vi "new destination folder for pictures.vi"(7 "scanners[]":string[](array[string]), 8 "error in":errorcluster, 10 "Info":T1={"Make"="", "Model"="", "Orientation"=0, "Date"=timestamp(0 s since 1904-01-01), "Width"=0, "Height"=0, "Square?"=FALSE, "File Name"="", "Extension"="", "Valid?"=FALSE, "Path"=path "", "size"=0, "No Ext?"=FALSE, "prefix?"=FALSE, "String"="", "Name Type"=enum."Event Sufix"}, 11 "dest path":path) -> (0 "error out":errorcluster, 3 "new dest filder path":path)   [LabVIEW 2023, in "File Classes.lvlib" / "Picture File.lvclass"]
uses:
  Picture File.lvclass
  Controls/exif data cluster.ctl
  Controls/rename type enum.ctl
  File Classes.lvlib
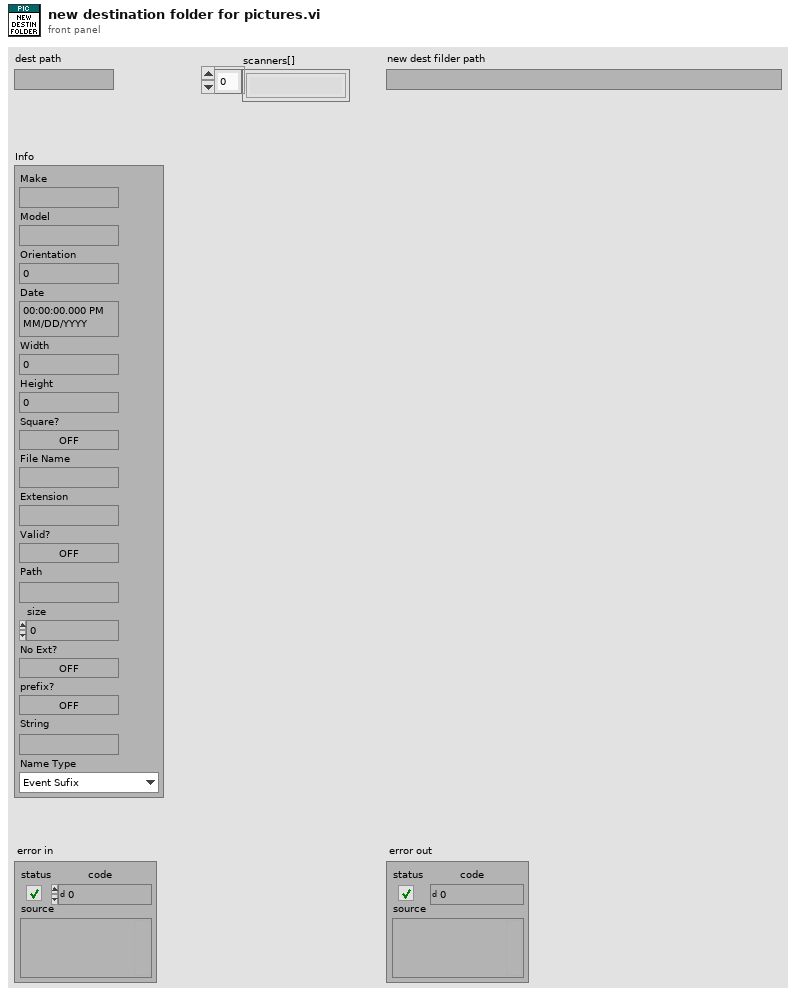
[diagram p1: front panel]
types:
  T1 = typedef "File Classes.lvlib/exif data cluster.ctl" = cluster{"Make":string, "Model":string, "Orientation":u16, "Date":timestamp, "Width":u16, "Height":u16, "Square?":bool, "File Name":string, "Extension":string, "Valid?":bool, "Path":path, "size":i64, "No Ext?":bool, "prefix?":bool, "String":string, "Name Type":T2}
  T2 = typedef "File Classes.lvlib/rename type enum.ctl" = enum16{"Date & Time (Default)", "Model Sufix", "Event Sufix", "Model & Event Sufix"}
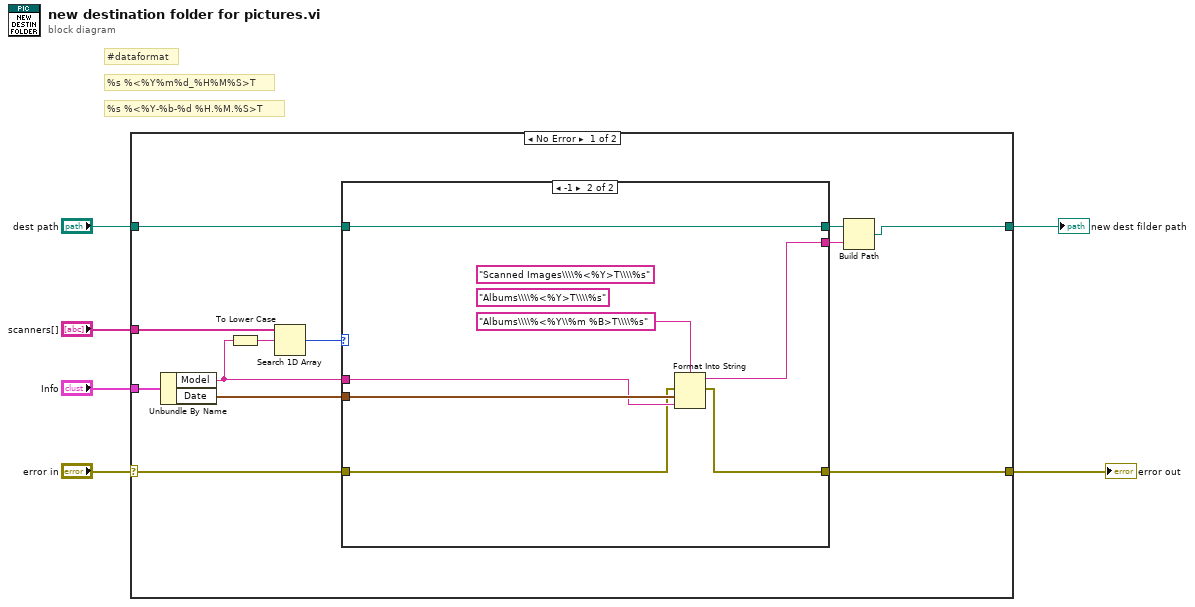
[diagram p0: block diagram]
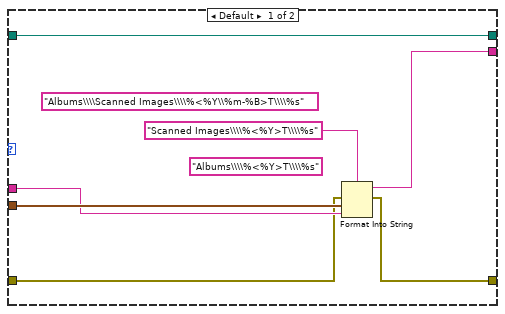
[diagram p2: hidden frame]
diagram:
  # "#dataformat"
  # "%s %<%Y-%b-%d %H.%M.%S>T"
  # "%s %<%Y%m%d_%H%M%S>T"
  n1 = case shown="No Error" "error in" {
    selector: "error in" -> [w12 w33]
    tunnel: "scanners[]" -> [w18 _]
    tunnel: "Info" -> [w16 _]
    tunnel: "dest path" -> [w13 w34]
    tunnel: [w8 w34] -> w3
    tunnel: [w7 w33] -> w2
    frame No Error {
      n2 = Unbundle By Name(w16) -> ("Model"=w11:string, "Date"=w9:timestamp)
      n3 = To Lower Case(string=w11) -> (all lower case string=w17:string)
      n4 = Search 1D Array(1D array=w18, element=w17) -> (index of element=w15:i32)  [unwired: 1 in]
      n5 = case shown="-1" w15 {
        tunnel: [w25 w32] -> w14
        tunnel: w13 -> [w25 w32]
        tunnel: [w21 w28] -> w7
        tunnel: w12 -> [w20 w27]
        tunnel: w11 -> [w23 w30]
        tunnel: [w22 w29] -> w10
        tunnel: w9 -> [w24 w31]
        frame Default {
          (unwired) "Albums\\\\Scanned Images\\\\%<%Y\\%m-%B>T\\\\%s" ("format string")
          (unwired) "Albums\\\\%<%Y>T\\\\%s" ("format string")
          n6 = Format Into String(format string="Scanned Images\\\\%<%Y>T\\\\%s", error in=w20, w24, w23) -> (resulting string=w22:string, error out=w21:errorcluster)  [unwired: 1 in]
        }
        frame -1 {
          (unwired) "Albums\\\\%<%Y>T\\\\%s" ("format string")
          (unwired) "Scanned Images\\\\%<%Y>T\\\\%s" ("format string")
          n7 = Format Into String(format string="Albums\\\\%<%Y\\%m %B>T\\\\%s", error in=w27, w31, w30) -> (resulting string=w29:string, error out=w28:errorcluster)  [unwired: 1 in]
        }
      }
      n8 = Build Path(base path=w14, name or relative path=w10) -> (appended path=w8:path)
    }
    frame Error {
    }
  }
  "new dest filder path" <- w3
  "error out" <- w2
